vi "uTTA_ucf_WriteValue.vi"(5 "key":string, 6 "Value IN":dbl, 7 "section":string, 8 "error in (no error)":errorcluster, 11 "ucf-FileRef in":T1) -> (0 "error out":errorcluster, 3 "ucf-FileRef out":T1)   [LabVIEW 2021]
uses:
  <vilib>/Utility/config.llb/Config Data RefNum.ctl
  <vilib>/Utility/config.llb/Write Key (String).vi
  <vilib>/Utility/config.llb/NI_LVConfig.lvlib
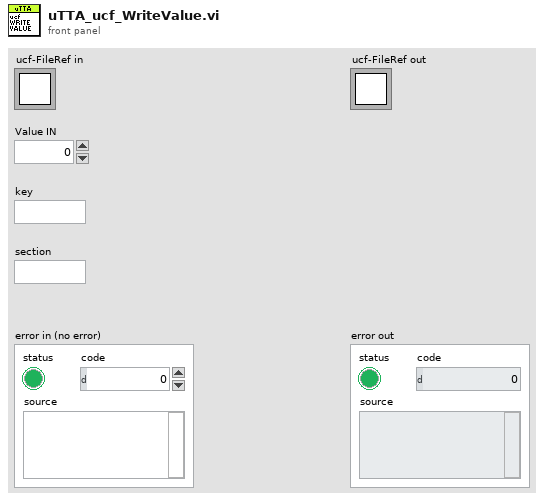
[diagram p1: front panel]
types:
  T1 = typedef "NI_LVConfig.lvlib/Config Data RefNum.ctl" = refnum<k1>
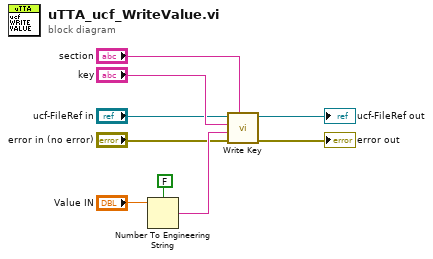
[diagram p0: block diagram]
diagram:
  n1 = Number To Engineering String(1:FALSE ("use system decimal point (T)"), 4:"Value IN") -> (0:w7:string)  [unwired: 2 in]
  n2 = call-poly <vilib>:"Write Key.vi"("section"="section", "error in (no error)"="error in (no error)", "value"=w7, "key"="key", "refnum"="ucf-FileRef in") -> ("error out"=→"error out":errorcluster, "refnum out"=→"ucf-FileRef out":T1)  [unwired: 4 in, 1 out]
